vi "test double click event.vi"() -> ()   [LabVIEW 2017]
panel:
  out "double click 2":timestamp
  out "String":string
  out "double click":timestamp
  in  "Boolean":bool
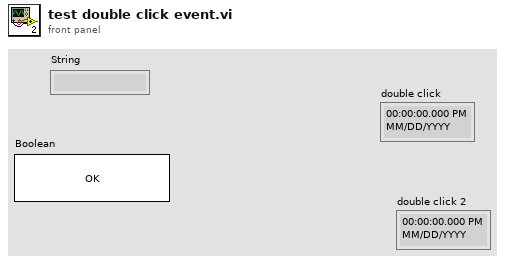
[diagram p1: front panel]
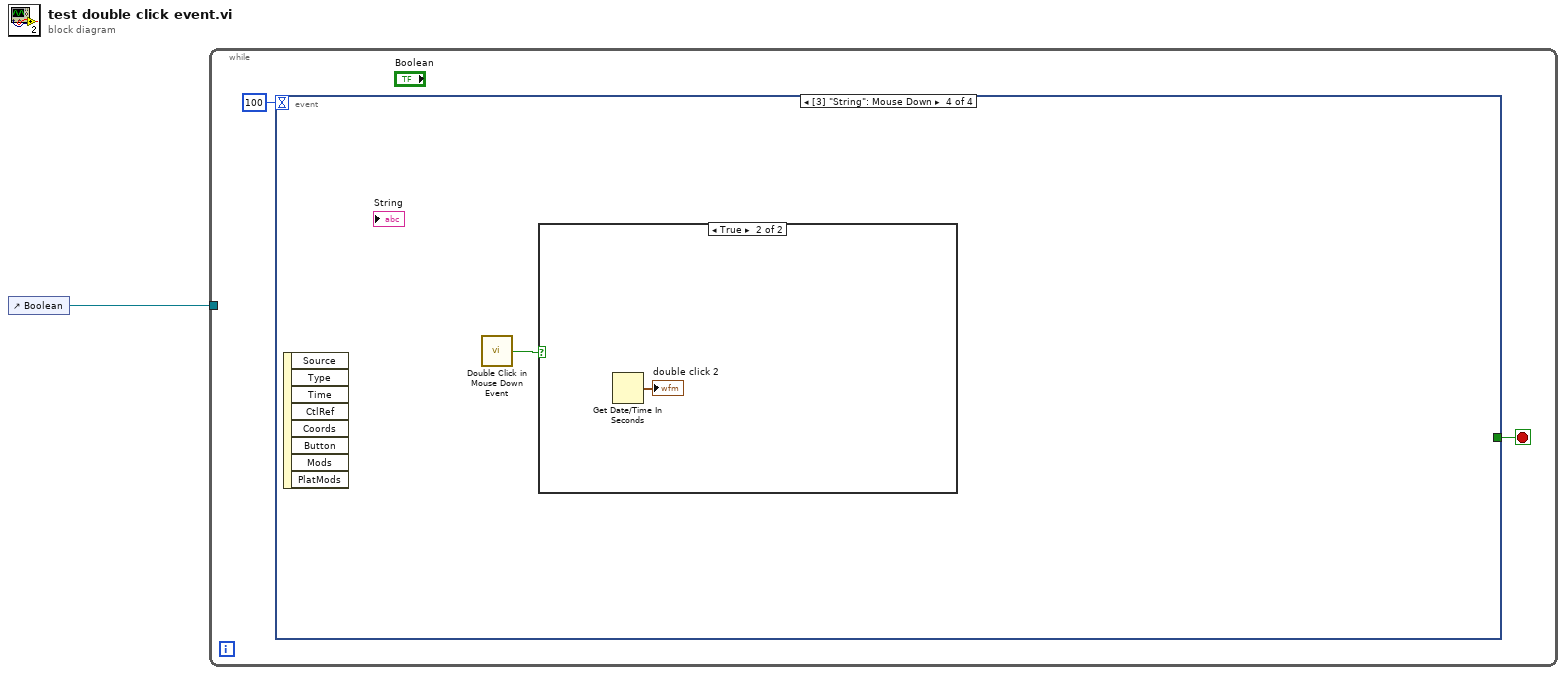
[diagram p0: block diagram]
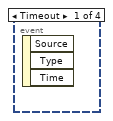
[diagram p2: hidden frame]
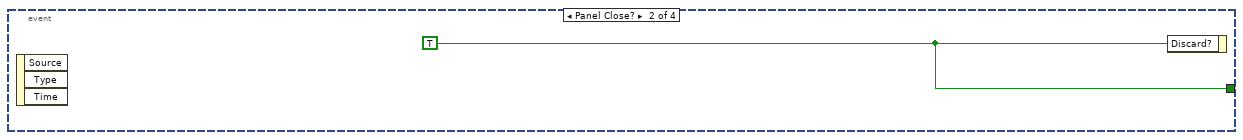
[diagram p3: hidden frame]
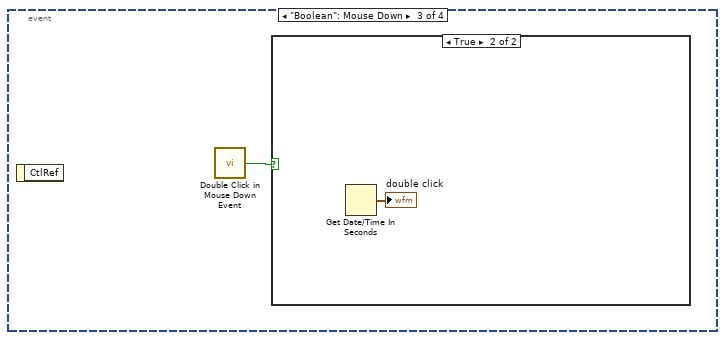
[diagram p4: hidden frame]
diagram:
  n1 = control-ref of="Boolean"() -> (w1:refnum<vi>)
  n2 = while {
    tunnel: w1 -> [_]
    stop <- w3 stop-if-true
    n3 = event shown="[3] \"String\": Mouse Down" {
      selector: _ -> [_ _ _ _]
      dyn-events: _ -> [_ _ _ _]
      timeout: 100 -> [_ _ _ _]
      tunnel: [_ w4 _ _] -> w3
      event Timeout {
        n4 = event-data() -> ()  [unwired: 1 in, 3 out]
      }
      event Panel Close? {
        w4 = TRUE ("Discard?")
        n5 = event-data() -> ()  [unwired: 1 in, 3 out]
        n6 = event-data("Discard?"=w4) -> ()  [unwired: 1 in, 1 out]
      }
      event "Boolean": Mouse Down {
        n7 = event-data() -> ()  [unwired: 1 in, 1 out]
        n8 = call "Double Click in Mouse Down Event.vi"() -> ("Double Click?"=w5:bool)  [unwired: 5 in]
        n9 = case shown="True" w5 {
          frame False {
          }
          frame True {
            n10 = Get Date/Time In Seconds() -> (seconds since 1Jan1904=→"double click":timestamp)
          }
        }
      }
      event "String": Mouse Down {
        n11 = event-data() -> ()  [unwired: 1 in, 8 out]
        n12 = call "Double Click in Mouse Down Event.vi"() -> ("Double Click?"=w7:bool)  [unwired: 5 in]
        n13 = case shown="True" w7 {
          frame False {
          }
          frame True {
            n14 = Get Date/Time In Seconds() -> (seconds since 1Jan1904=→"double click 2":timestamp)
          }
        }
      }
    }
  }
